vi "WaitOnErrorNotifier.vi"(8 "error in (no error)":errorcluster, 9 "Timeout additional message (\"\")":string, 10 "Timeout [ms]":i32, 11 "Error Notifier":refnum<notifier>) -> (0 "error out":errorcluster)   [LabVIEW 2020, in "GLF.lvlib" / "Engine.lvclass"]
uses:
  Engine.lvclass
  Engine.lvclass/Engine.ctl
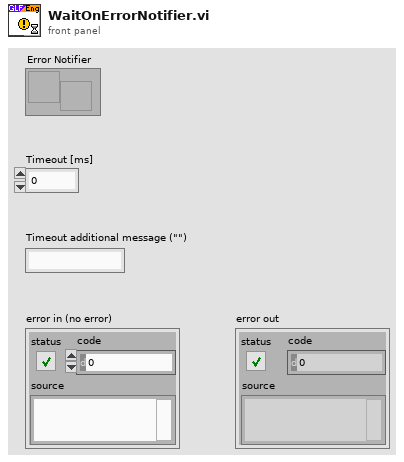
[diagram p1: front panel]
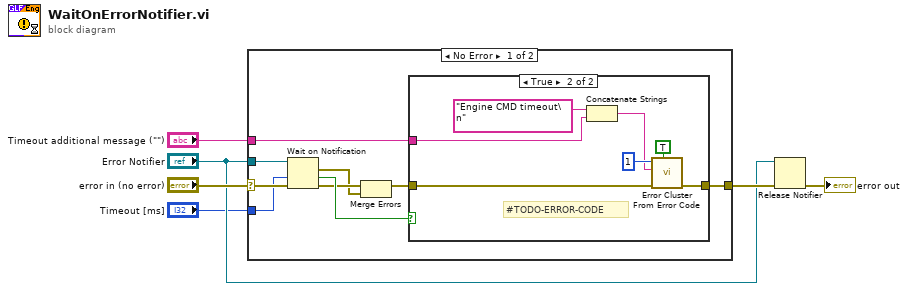
[diagram p0: block diagram]
diagram:
  n1 = case shown="No Error" "error in (no error)" {
    selector: "error in (no error)" -> [w13 w24]
    tunnel: [w12 w24] -> w5
    tunnel: "Error Notifier" -> [w11 _]
    tunnel: "Timeout [ms]" -> [w9 _]
    tunnel: "Timeout additional message (\"\")" -> [w8 _]
    frame No Error {
      n2 = Wait on Notification(notifier=w11, timeout in ms (-1)=w9, error in (no error)=w13) -> (notification=w7:errorcluster, timed out?=w14:bool, error out=w10:errorcluster)  [unwired: 1 in, 1 out]
      n3 = Merge Errors(w10, w7) -> (w15:errorcluster)
      n4 = case shown="True" w14 {
        tunnel: w15 -> [w16 w23]
        tunnel: [w16 w22] -> w12
        tunnel: w8 -> [_ w17]
        frame False {
        }
        frame True {
          # "#TODO-ERROR-CODE"
          n5 = Concatenate Strings("Engine CMD timeout\n" ("error message (\"\")"), w17) -> (w18:string)
          n6 = call <vilib>:"Error Cluster From Error Code.vi"("show call chain? (False)"=TRUE, "error in (no error)"=w23, "error message (\"\")"=w18, "error code (0)"=1) -> ("error out"=w22:errorcluster)  [unwired: 5 in]
        }
      }
    }
    frame Error {
    }
  }
  n7 = Release Notifier(notifier="Error Notifier", error in (no error)=w5) -> (error out=→"error out":errorcluster)  [unwired: 1 in, 2 out]
